vi "ReadWrite.Close.vi"(8 "error in":errorcluster, 11 "ReadWrite in":refnum<class "ReadWrite.lvclass">) -> (0 "error out":errorcluster, 3 "ReadWrite out":refnum<class "ReadWrite.lvclass">)   [LabVIEW 2026, in "Data Access Engine (Express).lvlib" / "ReadWrite.lvclass"]
uses:
  ReadWrite.lvclass
  ReadWrite.lvclass/ReadWrite.ctl
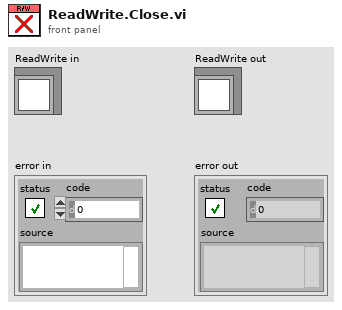
[diagram p1: front panel]
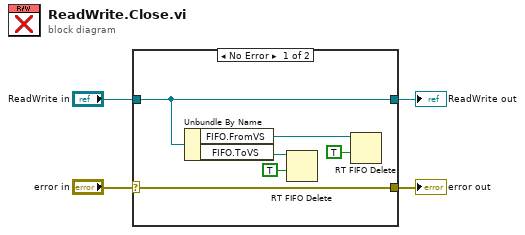
[diagram p0: block diagram]
diagram:
  n1 = case shown="No Error" "error in" {
    selector: "error in" -> [w10 w12]
    tunnel: [w10 w12] -> w3
    tunnel: [w7 w11] -> w1
    tunnel: "ReadWrite in" -> [w7 w11]
    frame No Error {
      n2 = Unbundle By Name(w7) -> ("FIFO.FromVS"=w5:refnum<k33>, "FIFO.ToVS"=w9:refnum<k33>)
      n3 = RT FIFO Delete(0:w9, 2:TRUE ("force destroy? (F)")) -> ()  [unwired: 1 in, 1 out]
      n4 = RT FIFO Delete(0:w5, 2:TRUE ("force destroy? (F)")) -> ()  [unwired: 1 in, 1 out]
    }
    frame Error {
    }
  }
  "error out" <- w3
  "ReadWrite out" <- w1
